vi "write flicker file.vi"(1 "Array":string[](array[string]), 2 "Waveform Data":waveform(dbl), 3 "appended path":path) -> ()   [LabVIEW 2013]
uses:
  <vilib>/Waveform/WDTOps.llb/WDT Waveform Duration DBL.vi
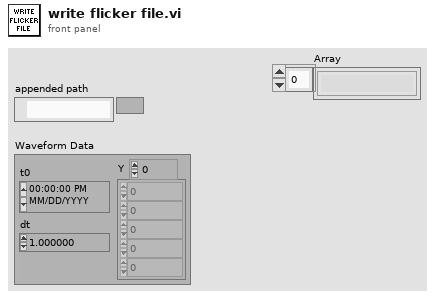
[diagram p1: front panel]
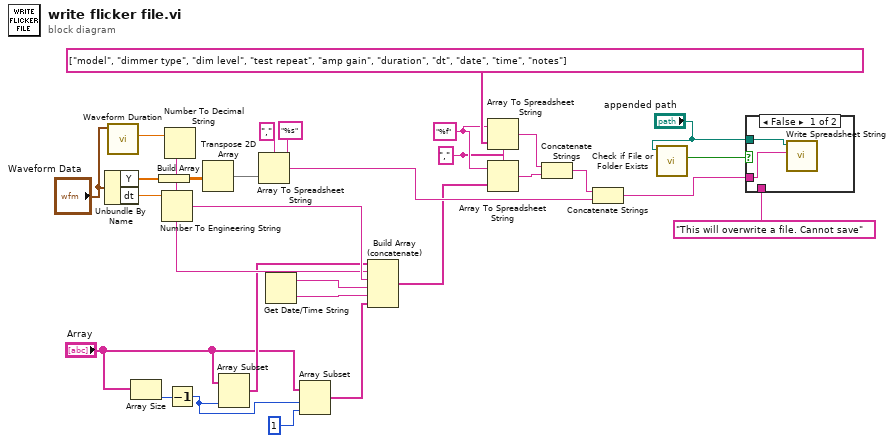
[diagram p0: block diagram]
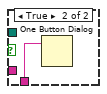
[diagram p2: hidden frame]
diagram:
  w5 = "," ("delimiter (Tab)")
  w19 = "%f" ("format string")
  n1 = Unbundle By Name("Waveform Data") -> ("Y"=w26:dbl[], "dt"=w17:dbl)
  n2 = call-poly <vilib>:"Waveform Duration.vi"("waveform in"="Waveform Data") -> ("duration"=w13:dbl)  [unwired: 8 in, 2 out]
  n3 = Array Size(array="Array") -> (size(s)=w9:i32)
  n4 = Build Array(w26) -> (w29:dbl[][])
  n5 = Number To Engineering String(4:w17) -> (0:w18:string)  [unwired: 3 in]
  n6 = Number To Decimal String(number=w13) -> (decimal integer string=w12:string)  [unwired: 1 in]
  n7 = Decrement(x=w9) -> (x-1=w6:i32)
  n8 = Transpose 2D Array(2D array=w29) -> (transposed array=w25:dbl[][])
  n9 = Array Subset(array="Array", length=w6) -> (w11:string[])  [unwired: 1 in]
  n10 = Array To Spreadsheet String(delimiter (Tab)=",", array=w25, 3:"%s" ("format string")) -> (spreadsheet string=w27:string)
  n11 = Get Date/Time String() -> (date string=w16:string, time string=w15:string)  [unwired: 3 in]
  n12 = Array Subset(array="Array", index=w6, length=1) -> (w7:string[])
  n13 = Build Array (concatenate)(w11, w12, w18, w16, w15, w7) -> (w14:string[])
  n14 = Array To Spreadsheet String(delimiter (Tab)=w5, array=string[] ["model", "dimmer type", "dim level", "test repeat", "amp gain", "duration", "dt", "date", "time", "notes"], 3:w19) -> (spreadsheet string=w21:string)
  n15 = Array To Spreadsheet String(delimiter (Tab)=w5, array=w14, 3:w19) -> (spreadsheet string=w24:string)
  n16 = Concatenate Strings(w21, w24) -> (w23:string)
  n17 = Concatenate Strings(w23, w27) -> (w1:string)
  n18 = call <vilib>:"Check if File or Folder Exists.vi"("path"="appended path") -> ("file or folder exists?"=w4:bool)  [unwired: 8 in, 2 out]
  n19 = case shown="False" w4 {
    tunnel: "appended path" -> [w32 _]
    tunnel: "This will overwrite a file. Cannot save" ("message") -> [_ w33]
    tunnel: w1 -> [w31 _]
    frame False {
      n20 = call <vilib>:"Write Spreadsheet String.vi"("spreadsheet string"=w31, "file path (dialog if empty)"=w32) -> ()  [unwired: 8 in, 2 out]
    }
    frame True {
      n21 = One Button Dialog(message=w33) -> ()  [unwired: 1 in, 1 out]
    }
  }
